vi "Program_Active_Aborting.vi"() -> ()   [LabVIEW 2010]
doc: "This is an example of using features of the VI Server as a client. It shows how you might browse from one or more applications that may be exporting data from one or more data stations. \n\nThe example shows how to query a server for its list of exported VIs, how to get references to the VIs, and how call them with the Call By Reference function."
uses:
  Sub VIs/ADAM Controls/Traverse_Level_State.ctl
  Anemometry/Anemometry Sub Vis/Globals/Preference_global.vi
  Anemometry/Anemometry Sub Vis/Globals/Meas_global.vi
  Anemometry/Anemometry Sub Vis/Globals/Dynamic_call_global.ph.vi
panel:
  out "error out":errorcluster
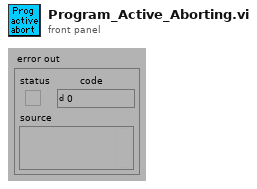
[diagram p1: front panel]
types:
  T1 = typedef "Server_Comms.ctl" = enum16{"Server Link Healthy", "Do Not Link To Server"}
  T2 = typedef "Traverse_Level_State.ctl" = enum16{"Running", "Complete"}
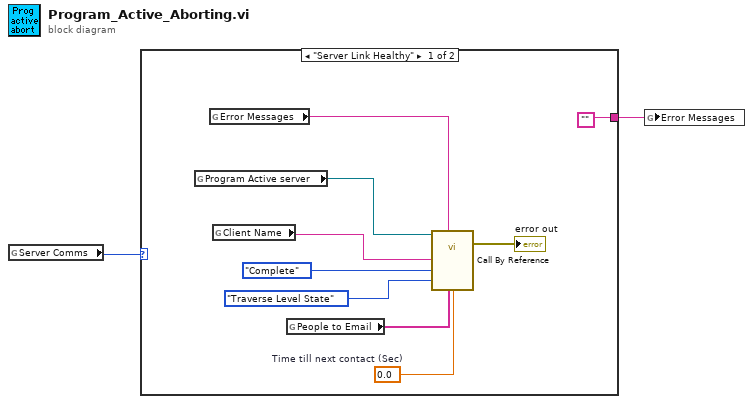
[diagram p0: block diagram]
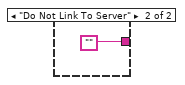
[diagram p2: hidden frame]
diagram:
  n1 = global read "Preference_global.vi" "Server Comms"() -> (w2:T1)
  n2 = case shown="\"Server Link Healthy\"" w2 {
    tunnel: ["" ""] -> w1
    frame "Server Link Healthy" {
      w3 = 0.0  # Time till next contact (Sec)
      n3 = global read "Dynamic_call_global.ph.vi" "Program Active server"() -> (w10:refnum<vi>)
      n4 = global read "Meas_global.vi" "Error Messages"() -> (w5:string)
      n5 = global read "Dynamic_call_global.ph.vi" "Client Name"() -> (w6:string)
      n6 = global read "Meas_global.vi" "People to Email"() -> (w11:string[])
      n7 = call-by-ref "?"(reference=w10, "Client Name"=w6, "Client Messages"=w5, "Traverse level State"=Traverse_Level_State."Complete", "Mode"=enum16{"Program Active", "Traverse Level State"}."Traverse Level State", "People to Email"=w11, "Time till next contact (Sec)"=w3) -> (error out=→"error out":errorcluster)  [unwired: 6 in, 1 out]
    }
    frame "Do Not Link To Server" {
    }
  }
  n8 = global write "Meas_global.vi" "Error Messages"(w1) -> ()
